vi "Create Filter.vi"(8 "error in (no error)":errorcluster, 11 "Session in":refnum<k21>="localhost") -> (0 "error out":errorcluster, 2 "Filter out":refnum<k20>, 3 "Session out":refnum<k21>)   [LabVIEW 2012, in "nisyscfg.lvlib"]
doc: "Creates a system filter object that is used to query for specific resources in a system. After creating a filter, set one or more properties using the Property Node (Filter) to limit the set of detected resources."
uses:
  <vilib>/nisyscfg/nisyscfg.lvlib
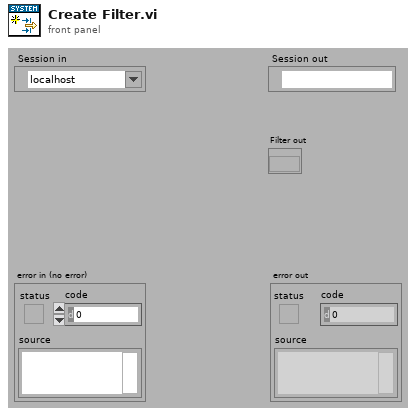
[diagram p1: front panel]
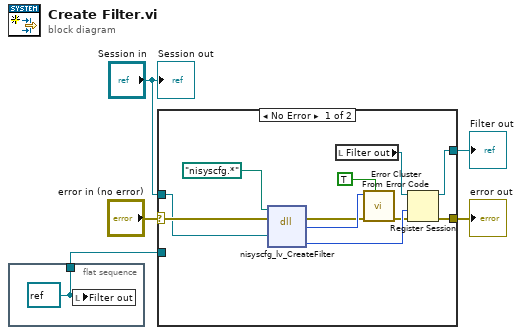
[diagram p0: block diagram]
diagram:
  n1 = flat-sequence {
    tunnel: [w6] -> w1
    frame #0 {
      w6 = refnum<k20> refnum ("filter out")
      n2 = local write "Filter out"(w6) -> ()
    }
  }
  n3 = case shown="No Error" "error in (no error)" {
    selector: "error in (no error)" -> [w11 w18]
    tunnel: [w13 w18] -> w5
    tunnel: "Session in" -> [w10 _]
    tunnel: [w12 _] -> w2
    tunnel: w1 -> [_ _]
    frame No Error {
      n4 = dll-call lib="nisyscfg.*" fn="nisyscfg_lv_CreateFilter" label="CreateFilter"(path in=path "nisyscfg.*", error in=w11, "framework"=w10) -> (error out=w16:errorcluster, "status"=w17:i32, "filter"=w15:u64)  [unwired: 1 in, 3 out]
      n5 = local read "Filter out"() -> (w7:refnum<k20>)
      n6 = call <vilib>:"Error Cluster From Error Code.vi"("show call chain? (False)"=TRUE, "error in (no error)"=w16, "error code (0)"=w17) -> ("error out"=w14:errorcluster)  [unwired: 6 out]
      n7 = Register Session(8:w14, 9:w15, 11:w7) -> (0:w13:errorcluster, 3:w12:refnum<k20>)  [unwired: 2 in]
    }
    frame Error {
    }
  }
  "error out" <- w5
  "Filter out" <- w2
  "Session out" <- "Session in"
